vi "TimeChannelStorage.vi"(2 "error in (no error)":errorcluster, 3 "Timing Channel Settings":T1[][](array[typedef]) {"FrontPanelTime" format="%.3p"; "Pulse width (s)" format="%.3p"; "Delay (s)" format="%.3p"}, 4 "Data Value Reference in":refnum<data-value>) -> (0 "error out":errorcluster)   [LabVIEW 2014]
uses:
  <vilib>/MDSplus/Classes/Tree_Class/Tree.lvclass
  Controls/TimingChannelSettings.ctl
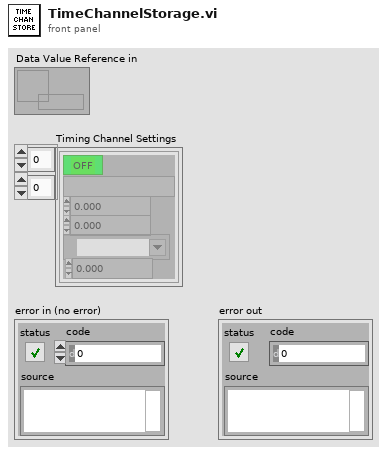
[diagram p1: front panel]
types:
  T1 = typedef "TimingChannelSettings.ctl" = cluster{"Delay (s)":dbl, "Pulse width (s)":dbl, "Active":bool, "Channel Name":string, "counter":tag, "FrontPanelTime":dbl}
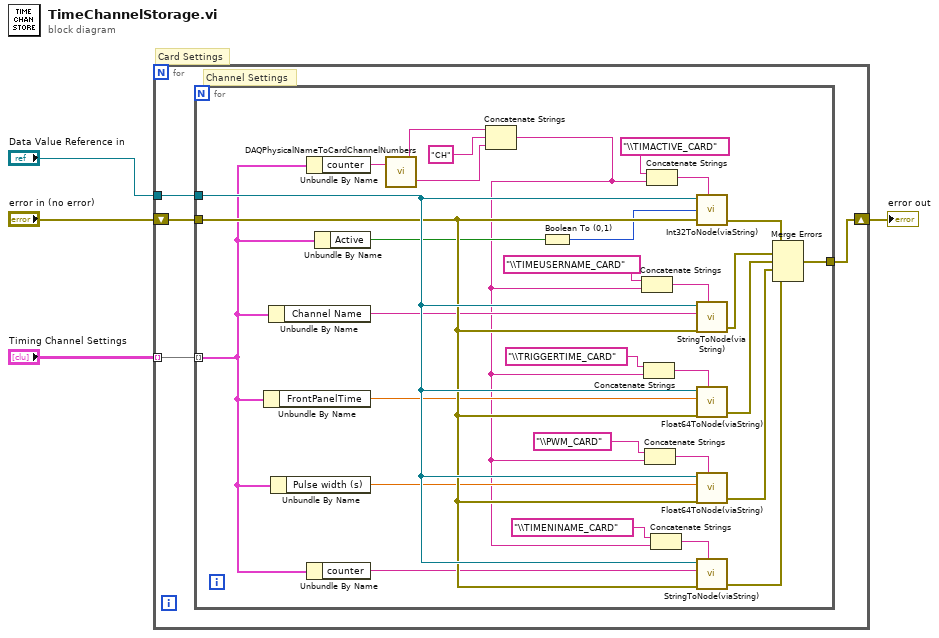
[diagram p0: block diagram]
diagram:
  # "Card Settings"
  n1 = for {
    shift-right: [w8] -> w1
    shift-left: "error in (no error)" -> [w6]
    tunnel: "Timing Channel Settings" -> [w7] mode=indexing
    tunnel: "Data Value Reference in" -> [w5]
    # "Channel Settings"
    n2 = for {
      tunnel: w7 -> [w35] mode=indexing
      tunnel: [w38] -> w8
      tunnel: w6 -> [w36]
      tunnel: w5 -> [w37]
      n3 = Unbundle By Name(w35) -> ("FrontPanelTime"=w23:dbl)
      n4 = Unbundle By Name(w35) -> ("Channel Name"=w29:string)
      n5 = Unbundle By Name(w35) -> ("Pulse width (s)"=w24:dbl)
      n6 = Unbundle By Name(w35) -> ("counter"=w17:tag)
      n7 = Unbundle By Name(w35) -> ("counter"=w25:tag)
      n8 = Unbundle By Name(w35) -> ("Active"=w31:bool)
      n9 = call "DAQPhysicalNameToCardChannelNumbers.vi"("NI Physical Channel"=w17) -> ("Channel #"=w15:string, "Card #"=w16:string)  [unwired: 1 in]
      n10 = Concatenate Strings(w16, "CH" ("string"), w15) -> (w10:string)
      n11 = Boolean To (0,1)(Boolean=w31) -> (0, 1=w33:i16)
      n12 = Concatenate Strings("\\TIMEUSERNAME_CARD" ("string"), w10) -> (w30:string)
      n13 = Concatenate Strings("\\TRIGGERTIME_CARD" ("string"), w10) -> (w28:string)
      n14 = Concatenate Strings("\\PWM_CARD" ("string"), w10) -> (w27:string)
      n15 = Concatenate Strings("\\TIMACTIVE_CARD" ("string"), w10) -> (w32:string)
      n16 = Concatenate Strings("\\TIMENINAME_CARD" ("string"), w10) -> (w26:string)
      n17 = call "Int32ToNode(viaString).vi"("Tree DVR in"=w37, "I32 in"=w33, "error in (no error)"=w36, "NodePath"=w32) -> ("error out"=w22:errorcluster)  [unwired: 3 in]
      n18 = call "StringToNode(viaString).vi"("Tree DVR in"=w37, "String value in"=w29, "error in (no error)"=w36, "NodePath"=w30) -> ("error out"=w21:errorcluster)  [unwired: 3 in]
      n19 = call "Float64ToNode(viaString).vi"("Tree DVR in"=w37, "DBL in"=w23, "error in"=w36, "NodePath"=w28) -> ("error out"=w20:errorcluster)  [unwired: 3 in]
      n20 = call "Float64ToNode(viaString).vi"("Tree DVR in"=w37, "DBL in"=w24, "error in"=w36, "NodePath"=w27) -> ("error out"=w19:errorcluster)  [unwired: 3 in]
      n21 = call "StringToNode(viaString).vi"("Tree DVR in"=w37, "String value in"=w25, "error in (no error)"=w36, "NodePath"=w26) -> ("error out"=w18:errorcluster)  [unwired: 3 in]
      n22 = Merge Errors(w22, w21, w20, w19, w18) -> (w38:errorcluster)
    }
  }
  "error out" <- w1
